vi "SSC Relay Control Core.vi"(0 "SSC Relay in":T1[](array[typedef]), 7 "Relay Commands":T2[](array[typedef]) items=["Open Relay"=20, "Close Relay"=21], 11 "error in":errorcluster) -> (4 "SSC Relay out":T1[](array[typedef]), 8 "Completed Relay Operations":T3[](array[typedef]) {"Desired State" items=["Open Relay"=20, "Close Relay"=21]}, 15 "error out":errorcluster)   [LabVIEW 2019]
doc: "This VI will apply the inputted Relay Commands to each Relay instrument session. \n\nThe Relay Commands input array can be of variable size. The actual commands will be automatically expanded and mapped based on the number Pins (filtered) in the Instrument Sessions.\n\nCases for when and how the Relay Commands array gets automatically expanded:\n-If the array is empty a substitute array of default type will be used and an error will be thrown\n-If the array has one element the it will be mapped to all sessions\n-If the array is an even multiple size of the number of sessions the array will be mapped multiple times (used to expand across sites)\n-If the array is not an even multiple size the array will still be mapped but an a warning will be emitted\n-If the array is the same size as the instrument sessions it will be mapped one-to-one.\n-If the array is larger than the instrument sessions it will be shortened and a warning will be emitted"
uses:
  SubVIs/TSM Relay Completed Operations.ctl
  <instrlib>/niSwitch/niSwitch.llb/niSwitch Relay Action.ctl
  SSC Relay.ctl
  <vilib>/Utility/error.llb/Error Cluster From Error Code.vi
  <instrlib>/niSwitch/niSwitch.llb/niSwitch Get Relay Position.vi
  <instrlib>/niSwitch/niSwitch.llb/niSwitch Relay Control.vi
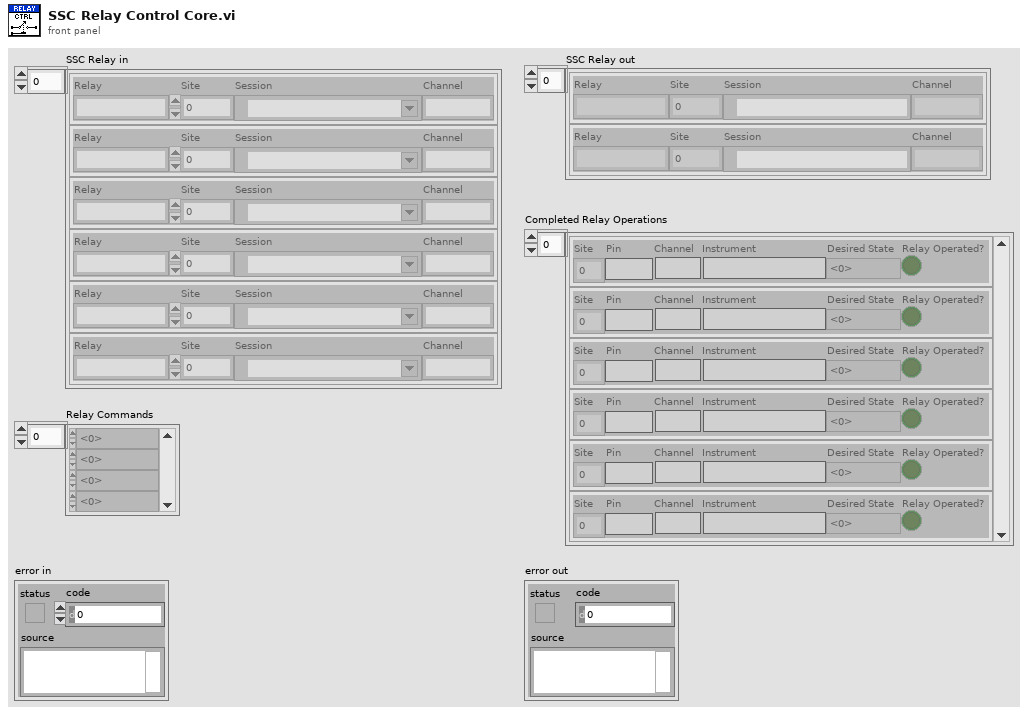
[diagram p1: front panel]
types:
  T1 = typedef "SSC Relay.ctl" = cluster{"Relay":string, "Site":i32, "Session":refnum<k15>, "Channel":string}
  T2 = typedef "niSwitch Relay Action.ctl" = i32
  T3 = typedef "TSM Relay Completed Operations.ctl" = cluster{"Site":i32, "Pin":string, "Channel":string, "Instrument":string, "Desired State":T2, "Relay Operated?":bool}
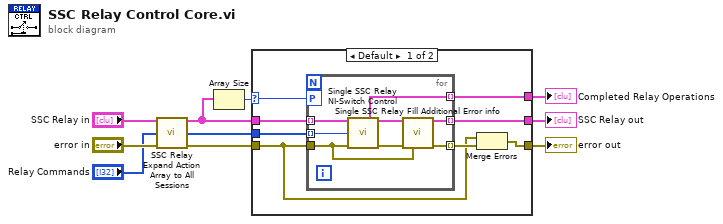
[diagram p0: block diagram]
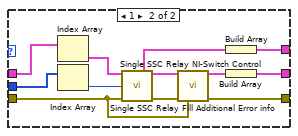
[diagram p2: hidden frame]
diagram:
  n1 = call "SSC Relay Expand Action Array to All Sessions.vi"("SSC Relay in"="SSC Relay in", "Relay Actions in"="Relay Commands", "error in"="error in") -> ("SSC Relay out"=w2:T1[], "Relay Actions out"=w3:T2[], "error out"=w6:errorcluster)  [unwired: 10 in]
  n2 = Array Size(array=w2) -> (size(s)=w9:i32)
  n3 = case shown="Default" w9 {
    selector: w9 -> [w14 _]
    tunnel: [w17 w29] -> w10
    tunnel: w6 -> [w16 w30]
    tunnel: [w15 w36] -> w8
    tunnel: w3 -> [w13 w35]
    tunnel: w2 -> [w12 w37]
    tunnel: [w11 w27] -> w1
    frame Default {
      n4 = for {
        tunnel: w16 -> [w23]
        tunnel: [w24] -> w18 mode=indexing
        workers-P: w14 -> [_]
        tunnel: [w20] -> w15 mode=indexing
        tunnel: w13 -> [w26] mode=indexing
        tunnel: w12 -> [w22] mode=indexing
        tunnel: [w19] -> w11 mode=indexing
        n5 = call "Single SSC Relay NI-Switch Control.vi"("SSC Relay in"=w22, "Operation"=w26, "error in"=w23) -> ("Completed Relay Operations"=w20:T3, "SSC Relay out"=w21:T1, "error out"=w25:errorcluster)  [unwired: 10 in]
        n6 = call "Single SSC Relay Fill Additional Error info.vi"("SSC Relay in"=w21, "error in"=w25, "previous error in"=w23) -> ("SSC Relay out"=w19:T1, "error out"=w24:errorcluster)  [unwired: 11 in]
      }
      n7 = Merge Errors(w16, w18) -> (w17:errorcluster)
    }
    frame 1 {
      n8 = Index Array(array=w37) -> (element=w38:T1)  [unwired: 1 in]
      n9 = Index Array(array=w35) -> (element=w34:T2)  [unwired: 1 in]
      n10 = call "Single SSC Relay NI-Switch Control.vi"("SSC Relay in"=w38, "Operation"=w34, "error in"=w30) -> ("Completed Relay Operations"=w33:T3, "SSC Relay out"=w31:T1, "error out"=w32:errorcluster)  [unwired: 10 in]
      n11 = call "Single SSC Relay Fill Additional Error info.vi"("SSC Relay in"=w31, "error in"=w32, "previous error in"=w30) -> ("SSC Relay out"=w28:T1, "error out"=w29:errorcluster)  [unwired: 11 in]
      n12 = Build Array(w33) -> (w36:T3[])
      n13 = Build Array(w28) -> (w27:T1[])
    }
  }
  "error out" <- w10
  "Completed Relay Operations" <- w8
  "SSC Relay out" <- w1
